vi "armBackDown.vi"(11 "putArmDown?":bool) -> ()   [LabVIEW 2013]
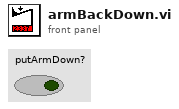
[diagram p1: front panel]
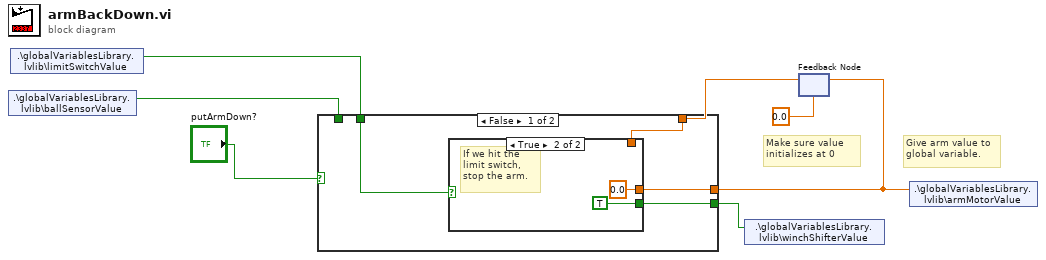
[diagram p0: block diagram]
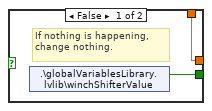
[diagram p2: hidden frame]
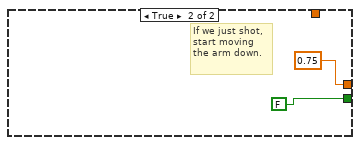
[diagram p3: hidden frame]
diagram:
  # "Make sure value initializes at 0"
  # "Give arm value to global variable."
  n1 = shared-variable ".\\globalVariablesLibrary.lvlib\\ballSensorValue"() -> (w2:bool)  [unwired: 1 in, 1 out]
  n2 = shared-variable ".\\globalVariablesLibrary.lvlib\\limitSwitchValue"() -> (w3:bool)  [unwired: 1 in, 1 out]
  n3 = feedback #1(0.0) -> (w5:dbl)
  n4 = case shown="False" "putArmDown?" {
    tunnel: [w11 0.75] -> w6
    tunnel: w5 -> [w10 _]
    tunnel: w3 -> [w9 _]
    tunnel: w2 -> [_ _]
    tunnel: [w8 FALSE] -> w1
    frame False {
      n5 = case shown="True" w9 {
        tunnel: [w13 0.0] -> w11
        tunnel: w10 -> [w13 _]
        tunnel: [w12 TRUE] -> w8
        frame False {
          # "If nothing is happening, change nothing."
          n6 = shared-variable ".\\globalVariablesLibrary.lvlib\\winchShifterValue"() -> (w12:bool)  [unwired: 1 in, 1 out]
        }
        frame True {
          # "If we hit the limit switch, stop the arm."
        }
      }
    }
    frame True {
      # "If we just shot, start moving the arm down."
    }
  }
  n7 = shared-variable ".\\globalVariablesLibrary.lvlib\\winchShifterValue"(w1) -> ()  [unwired: 1 in, 1 out]
  n8 = feedback-in #1(w6) -> ()
  n9 = shared-variable ".\\globalVariablesLibrary.lvlib\\armMotorValue"(w6) -> ()  [unwired: 1 in, 1 out]
